vi "Write Data (String).vi"(8 "error in (no error)":errorcluster, 10 "Write Buffer":string, 11 "Handle":u64) -> (0 "error out":errorcluster, 2 "Bytes Written":u32, 3 "Handle out":u64)   [LabVIEW 2019, in "D2XX-lv.lvlib"]
doc: "Write string data to the open device."
uses:
  D2XX-lv.lvlib
  <instrlib>/_D2XX/D2XX/D2XX.lvlib
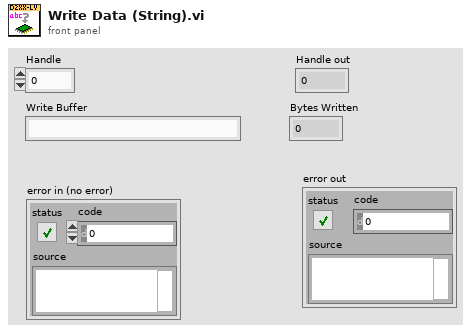
[diagram p1: front panel]
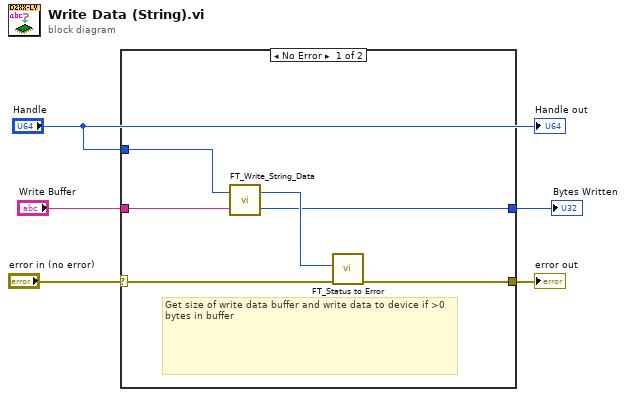
[diagram p0: block diagram]
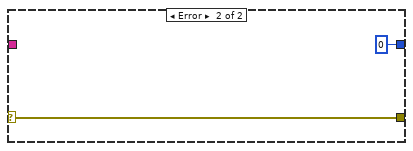
[diagram p2: hidden frame]
diagram:
  n1 = case shown="No Error" "error in (no error)" {
    selector: "error in (no error)" -> [w11 w13]
    tunnel: [w10 w13] -> w4
    tunnel: "Write Buffer" -> [w9 _]
    tunnel: "Handle" -> [w8 _]
    tunnel: [w6 u32 0 ("Bytes Written")] -> w1
    frame No Error {
      # "Get size of write data buffer and write data to device if >0 bytes in buffer"
      n2 = call <instrlib>:"FT_Write_String_Data.vi"("Buffer"=w9, "Handle"=w8) -> ("Bytes Written"=w6:u32, "FT_Status"=w7:u32)
      n3 = call "FT_Status to Error.vi"("error in (no error)"=w11, "FT_Status"=w7) -> ("error out"=w10:errorcluster)  [unwired: 9 in]
    }
    frame Error {
    }
  }
  "error out" <- w4
  "Bytes Written" <- w1
  "Handle out" <- "Handle"
